vi "Detect Mouse Move.vi"(10 "坐标":T1 caption="点32", 11 "窗格引用":refnum<vi>) -> (2 "Display[]":bool[](array[boolean]))   [LabVIEW 2016]
uses:
  <vilib>/Utility/miscctls.llb/LVPoint32TypeDef.ctl
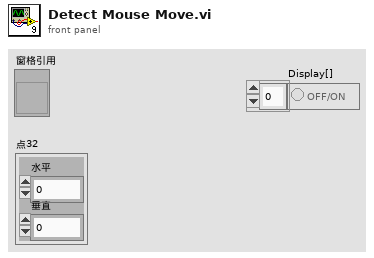
[diagram p1: front panel]
types:
  T1 = typedef "LVPoint32TypeDef.ctl" = cluster{"Horizontal":i32, "Vertical":i32}
  T2 = cluster{"top":i32, "buttom":i32, "left":i32, "right":i32, "Horizon Center":i32, "Vertical Center":i32}
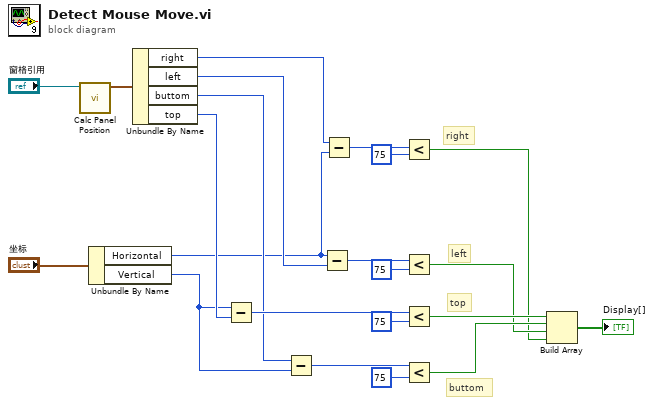
[diagram p0: block diagram]
diagram:
  # "buttom"
  # "top"
  # "right"
  # "left"
  n1 = call "Calc Panel Position.vi"("窗格引用"="窗格引用") -> ("Panel Position"=w7:T2)  [unwired: 10 in]
  n2 = Unbundle By Name("坐标") -> ("Horizontal"=w2:i32, "Vertical"=w1:i32)
  n3 = Unbundle By Name(w7) -> ("right"=w3:i32, "left"=w4:i32, "buttom"=w5:i32, "top"=w6:i32)
  n4 = Subtract(x=w1, y=w6) -> (x-y=w15:i32)
  n5 = Subtract(x=w5, y=w1) -> (x-y=w14:i32)
  n6 = Subtract(x=w2, y=w4) -> (x-y=w17:i32)
  n7 = Subtract(x=w3, y=w2) -> (x-y=w16:i32)
  n8 = Less?(x=w16, y=75) -> (x < y?=w10:bool)
  n9 = Less?(x=w17, y=75) -> (x < y?=w11:bool)
  n10 = Less?(x=w15, y=75) -> (x < y?=w13:bool)
  n11 = Less?(x=w14, y=75) -> (x < y?=w12:bool)
  n12 = Build Array(w13, w12, w11, w10) -> (→"Display[]":bool[])
